vi "Write Multiple rows.vi"(5 "Multiple rows":bool, 9 "Tab in":refnum<class "Tab.lvclass">) -> (3 "Tab out":refnum<class "Tab.lvclass">)   [LabVIEW 2014, in "Tab.lvclass"]
uses:
  Tab.lvclass
  Tab.lvclass/Tab.ctl
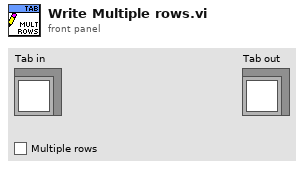
[diagram p1: front panel]
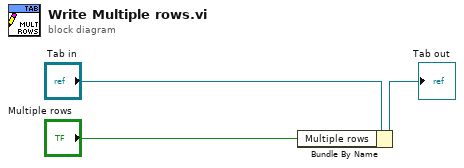
[diagram p0: block diagram]
diagram:
  n1 = Bundle By Name(cluster="Tab in", "Multiple rows"="Multiple rows") -> (→"Tab out":refnum<class "Tab.lvclass">)
